vi "EITDATA_SubFunctions.vi"() -> ()   [LabVIEW 2020]
doc: "This example demonstrates how to acquire a single buffer of voltage measurements using a DAQmx device.\n\nFor instructions on how to connect your signals to the DAQ device, refer to your device documentation."
uses:
  <vilib>/Utility/error.llb/DialogType.ctl
  <vilib>/DAQmx/read.llb/DAQmx Read (Analog 1D Wfm NChan NSamp).vi
  <vilib>/DAQmx/create/channels.llb/DAQmx Create Channel (AI-Voltage-Basic).vi
  <vilib>/DAQmx/configure/timing.llb/DAQmx Timing (Sample Clock).vi
  <vilib>/DAQmx/configure/trigger.llb/DAQmx Start Trigger (Digital Edge).vi
  <vilib>/DAQmx/configure/trigger.llb/DAQmx Start Trigger (Time).vi
  <vilib>/DAQmx/configure/trigger.llb/DAQmx Start Trigger (Analog Edge).vi
  <vilib>/DAQmx/configure/trigger.llb/DAQmx Reference Trigger (Digital Edge).vi
  <vilib>/DAQmx/configure/trigger.llb/DAQmx Reference Trigger (Analog Edge).vi
  <vilib>/DAQmx/miscellaneous.llb/DAQmx Fill In Error Info.vi
  <vilib>/express/express analysis/Spectral/Block/exnSpectralBlock spectral measurements PSD poly.vi
  <vilib>/express/express analysis/Spectral/Block/exnSpectralBlock spectral measurements PSD array WFM.vi
  <vilib>/express/express analysis/Spectral/XNode/ExpressSpectralMeasurementsBlockNode.xnode
  <resource>/objmgr/daqmx.rc
panel:
  out "Waveform Chart 2":dbl[](graph)
  out "looptime":dbl
  out "Waveform Graph 3":dbl[][](graph)
  in  "header text must have # at startr":string="#header text header text texty text text"
  out "Waveform Chart":T1(graph)
  in  "name or relative path":string="test.txt"
  in  "stop":bool
  out "Waveform Graph 2":cluster{"f0":dbl, "df":dbl, "magnitude":dbl[]}[](graph)
  in  "Trigger Type":T2(tab)
  in  "Digital Start Trigger Edge":i32(ring)=10280 caption="Edge" items=["Rising"=10280, "Falling"=10171]
  in  "Digital Start Trigger Source":tag="/Dev3/PFI0" caption="Source"
  in  "Digital Pause Trigger Pause When":i32(ring)=10192 caption="Pause When" items=["High"=10192, "Low"=10214]
  in  "Digital Pause Trigger Source":tag="/Dev1/PFI0" caption="Source"
  in  "Digital Reference Trigger Source":tag="/Dev1/PFI0" caption="Source"
  in  "Digital Reference Trigger Edge":i32(ring)=10280 caption="Edge" items=["Rising"=10280, "Falling"=10171]
  in  "Digital Reference Pretrigger Samples":u32 caption="Pretrigger Samples"
  in  "Analog Start Trigger Level":dbl caption="Level" format="%0.2f"
  in  "Analog Start Trigger Hysteresis":dbl caption="Hysteresis" format="%.2f"
  in  "Analog Start Trigger Slope":i32(ring)=10280 caption="Slope" items=["Rising"=10280, "Falling"=10171]
  in  "Analog Start Trigger Source":string="APFI0" caption="Source"
  in  "Analog Pause Trigger Source":string="APFI0" caption="Source"
  in  "Analog Pause Trigger Pause When":i32(ring)=10093 caption="Pause When" items=["Above Level"=10093, "Below Level"=10107]
  in  "Analog Pause Trigger Level":dbl caption="Level" format="%.2f"
  in  "Analog Reference Trigger Source":string="APFI0" caption="Source"
  in  "Analog Reference Trigger Level":dbl caption="Level" format="%.2f"
  in  "Analog Reference Trigger Slope":i32(ring)=10280 caption="Slope" items=["Rising"=10280, "Falling"=10171]
  in  "Analog Reference Pretrigger Samples":u32 caption="Pretrigger Samples"
  in  "When":timestamp
  in  "Select Time\nManually":bool
  out "Waveform Graph":waveform(dbl)[](graph)
  in  "Number of Samples":i32=1000
  in  "Sample Rate":dbl=50000.0
  in  "Sample Clock Source":tag="OnboardClock"
  in  "Terminal Configuration":i32(ring)=10083 items=["default"=-1, "RSE"=10083, "NRSE"=10078, "Differential"=10106, "Pseudodifferential"=12529]
  in  "Max Voltage":dbl=1.0
  in  "Min Voltage":dbl=-1.0
  in  "Physical Channel":tag="Dev3/ai0:15"
  out "Actual Sample Rate":dbl=1000.0 format="%0.2f"
  # "TIMEOUT AFTERWARDS IS NORMAL!!!!"
  # "Channel Settings"
  # "Acquired Data"
  # "Timing Settings"
  # "Trigger Settings"
  # "To enable triggers, select a tab above, and configure the settings.\n\nNot all hardware supports all trigger types. Refer to your device documentation for more information."
  # "If time is not manually set, task will begin after 10 seconds"
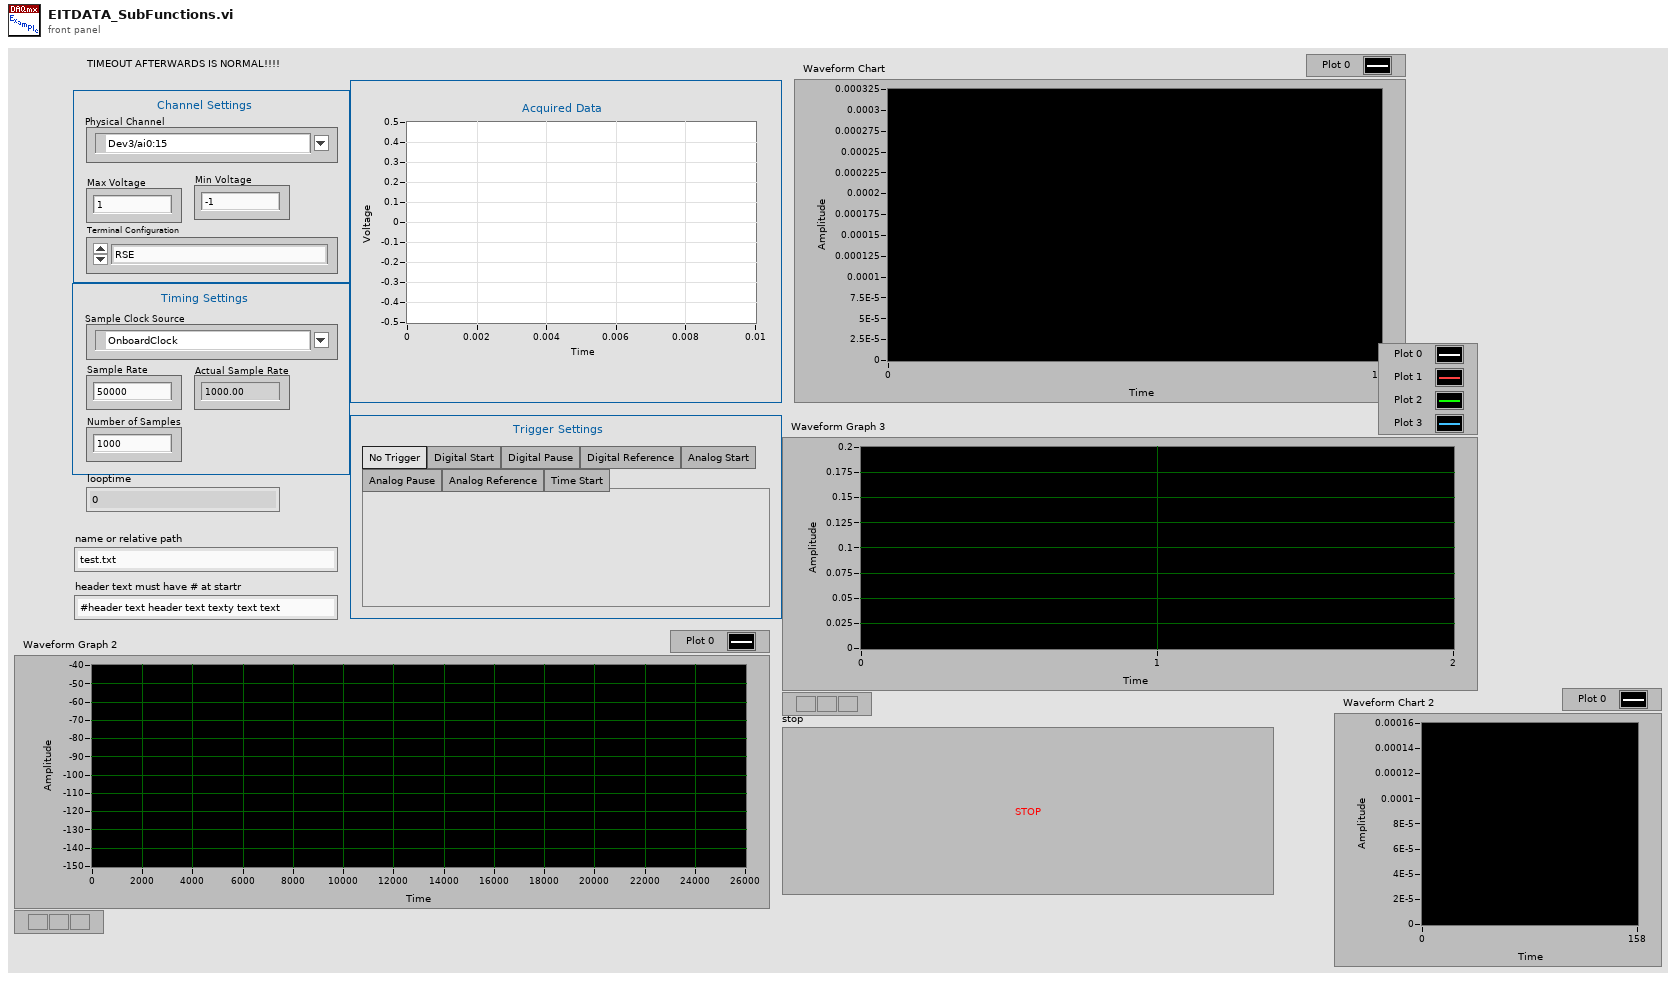
[diagram p1: front panel]
types:
  T1 = cluster{"detected amplitudes[0]":dbl, "detected amplitudes[1]":dbl, "detected amplitudes[2]":dbl, "detected amplitudes[3]":dbl, "detected amplitudes[4]":dbl, "detected amplitudes[5]":dbl, "detected amplitudes[6]":dbl, "detected amplitudes[7]":dbl, "detected amplitudes[8]":dbl}
  T2 = enum32{"No Trigger", "Digital Start", "Digital Pause", "Digital Reference", "Analog Start", "Analog Pause", "Analog Reference", "Time Start"}
  T3 = cluster{"detected amplitudes[0]":dbl, "detected amplitudes[1]":dbl, "detected amplitudes[2]":dbl, "detected amplitudes[3]":dbl, "detected amplitudes[4]":dbl, "detected amplitudes[5]":dbl, "detected amplitudes[6]":dbl, "detected amplitudes[7]":dbl, "detected amplitudes[8]":dbl}[]
  T4 = enum16{"open", "replace", "create", "open or create", "replace or create", "replace or create with confirmation"}
  T5 = typedef "DialogType.ctl" = u16
  T6 = cluster{"averaging mode":u16, "weighting mode":u16, "number of averages":u32}
  T7 = cluster{"dB On (F)":bool, "unwrap phase (F)":bool, "convert to degree (F)":bool}
  T8 = cluster{"Amp1D[0]":dbl, "Amp1D[1]":dbl, "Amp1D[2]":dbl, "Amp1D[3]":dbl, "Amp1D[4]":dbl, "Amp1D[5]":dbl, "Amp1D[6]":dbl, "Amp1D[7]":dbl, "Amp1D[8]":dbl}
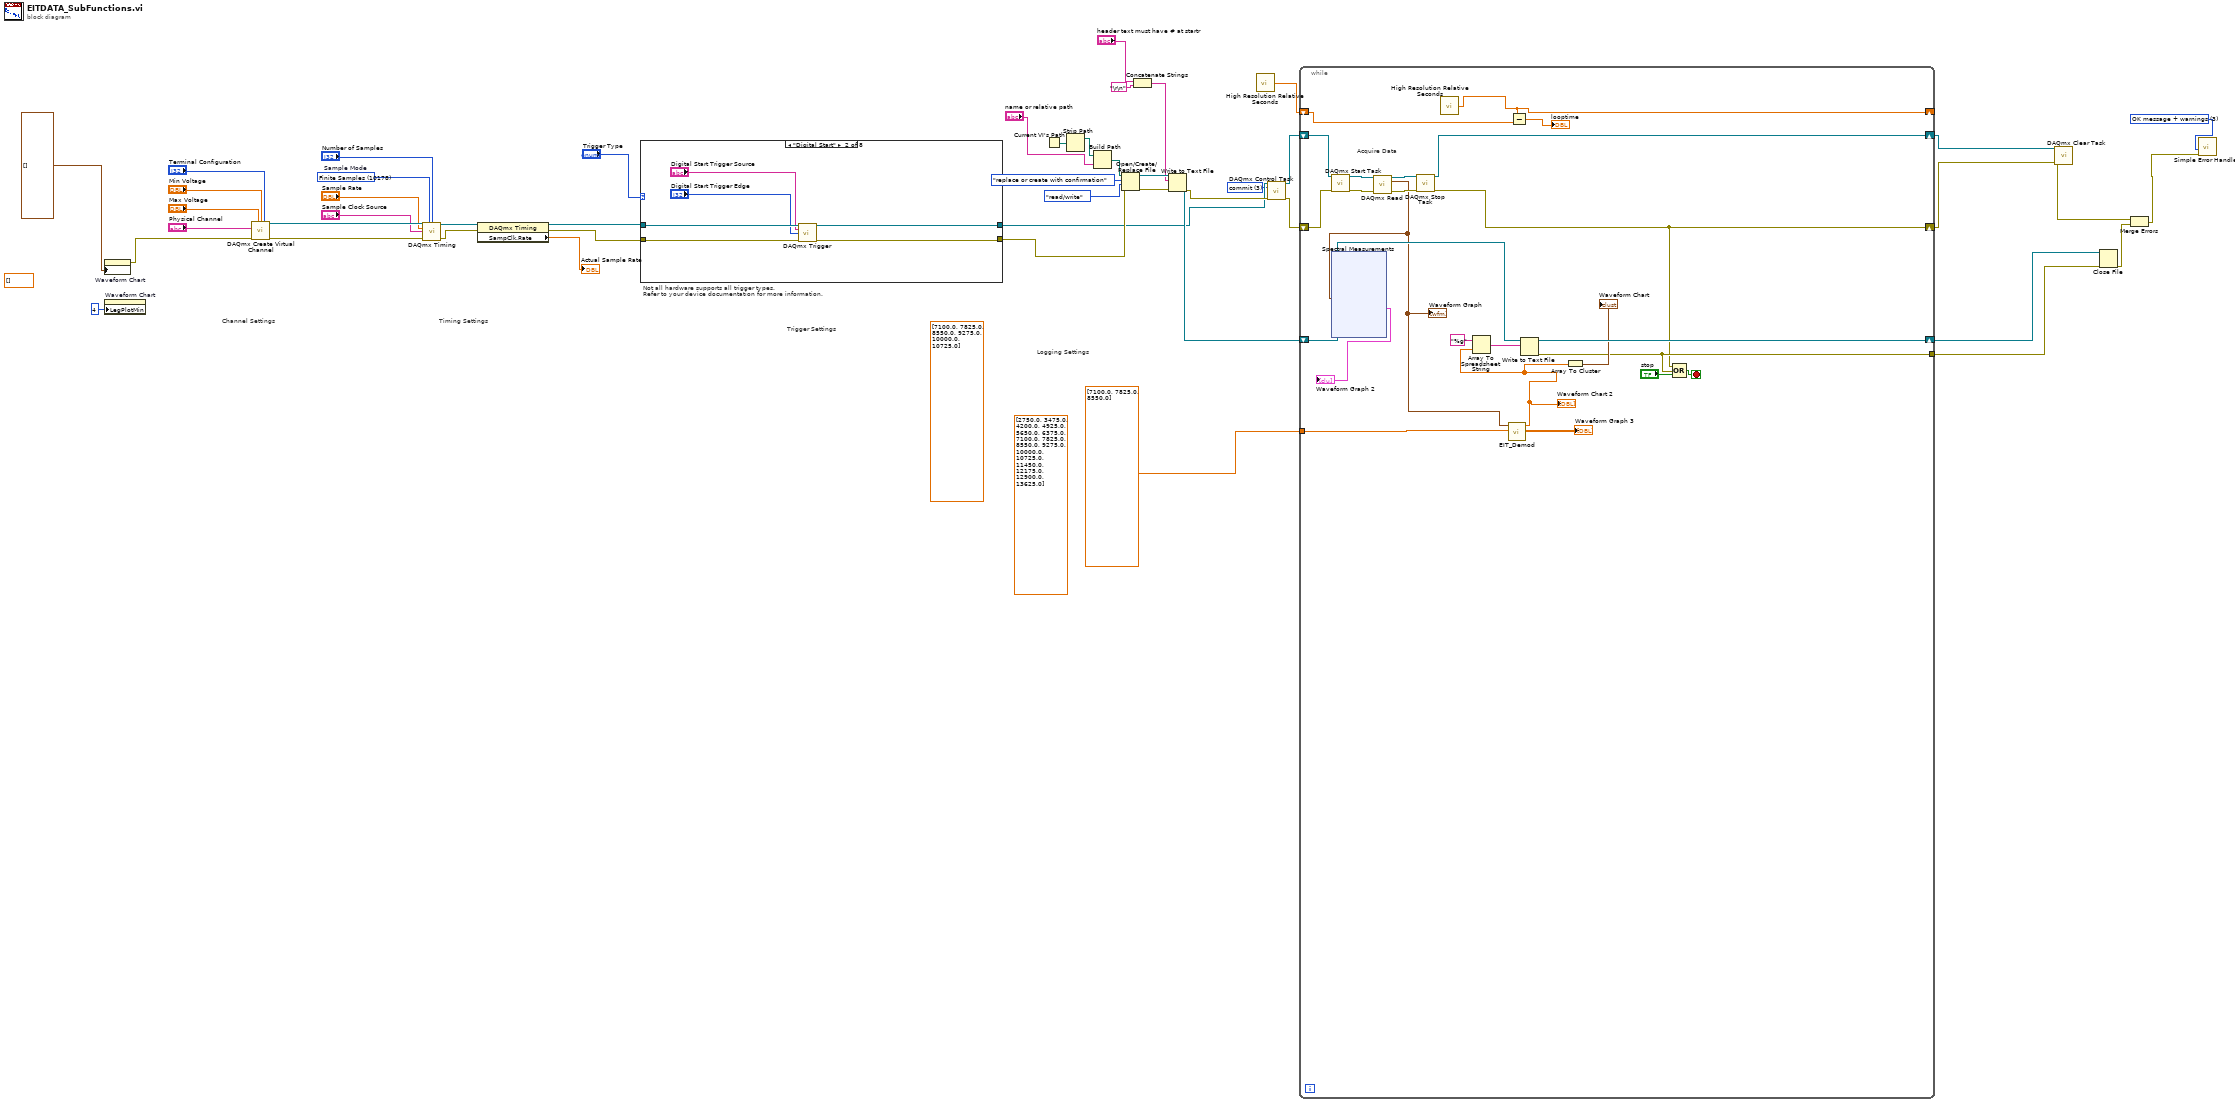
[diagram p0: block diagram]
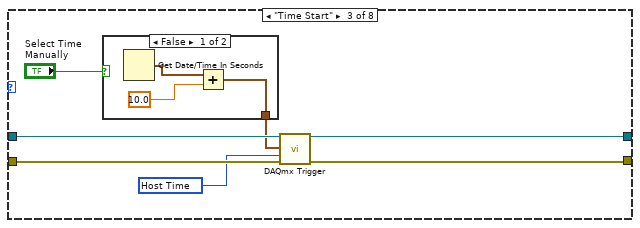
[diagram p3: hidden frame]
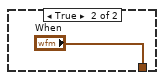
[diagram p4: hidden frame]
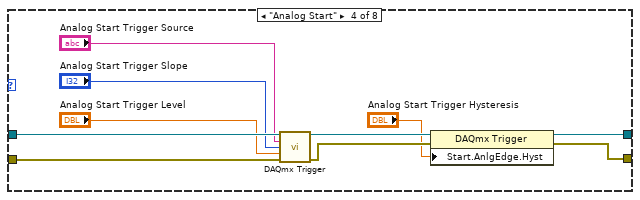
[diagram p5: hidden frame]
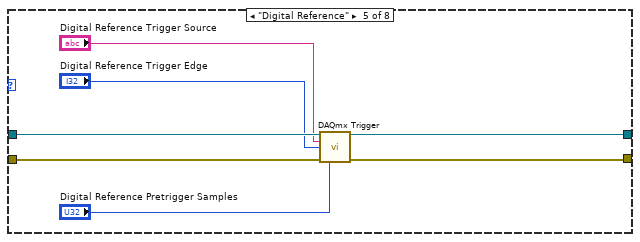
[diagram p6: hidden frame]
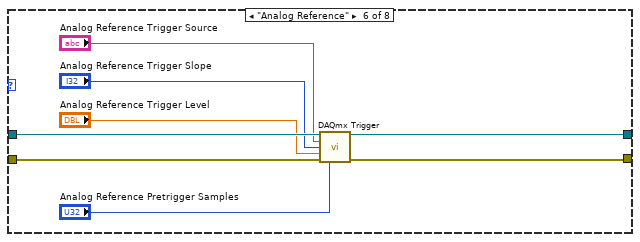
[diagram p7: hidden frame]
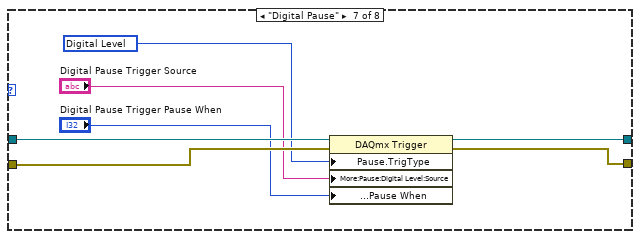
[diagram p8: hidden frame]
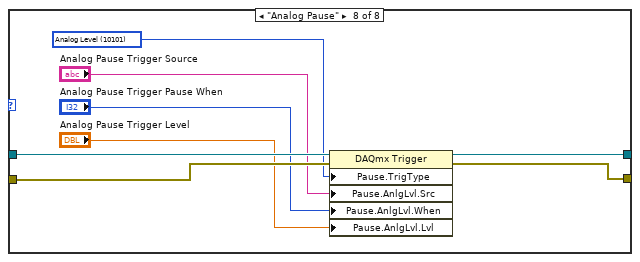
[diagram p9: hidden frame]
diagram:
  (unwired) dbl[] [7100.0, 7825.0, 8550.0, 9275.0, 10000.0, 10725.0]
  (unwired) dbl[] [2750.0, 3475.0, 4200.0, 4925.0, 5650.0, 6375.0, 7100.0, 7825.0, 8550.0, 9275.0, 10000.0, 10725.0, 11450.0, 12175.0, 12900.0, 13625.0]
  (unwired) dbl[] [] ("History Data")
  w12 = 3 items=["verify"=2, "reserve"=4, "commit"=3, "unreserve"=5, "abort"=6] ("action")
  w34 = T5 3 items=["no dialog", "OK message", "continue or stop message", "OK message + warnings", "continue/stop + warnings"] ("type of dialog (OK msg:1)")
  w45 = 10178 items=["Finite Samples"=10178, "Continuous Samples"=10123, "Hardware Timed Single Point"=12522]  # Sample Mode
  # "Not all hardware supports all trigger types.\nRefer to your device documentation for more information."
  # "Trigger Settings"
  # "Timing Settings"
  # "Channel Settings"
  # "Logging Settings"
  n1 = property on="Waveform Chart" class="WFChart (strict)"("History Data"=T3 []) -> (error out=w6:errorcluster)  [unwired: 2 in, 1 out]
  n2 = property on="Waveform Chart" class="WFChart (strict)"("LegPlotMin"=u32 4 ("Legend:Plot Minimum")) -> ()  [unwired: 2 in, 2 out]
  n3 = call-poly <vilib>:"DAQmx Create Virtual Channel.vi"("maximum value"="Max Voltage", "minimum value"="Min Voltage", "input terminal configuration"="Terminal Configuration", "physical channels"="Physical Channel", "error in"=w6) -> ("task out"=w43:refnum<k21>, "error out"=w44:errorcluster)  [unwired: 9 in]
  n4 = call-poly <vilib>:"DAQmx Timing.vi"("task/channels in"=w43, "sample mode"=w45, "samples per channel"="Number of Samples", "rate"="Sample Rate", "source"="Sample Clock Source", "error in"=w44) -> ("task out"=w47:refnum<k21>, "error out"=w46:errorcluster)  [unwired: 8 in]
  n5 = property class="DAQmx Timing"(reference=w47, error in=w46) -> (reference out=w31:refnum<k21>, error out=w32:errorcluster, "SampClk.Rate"=→"Actual Sample Rate":dbl)
  n6 = case shown="\"Digital Start\"" "Trigger Type" {
    tunnel: w31 -> [w49 w55 w62 w76 w83 w91 w98 w106]
    tunnel: w32 -> [w48 w54 w61 w75 w82 w90 w95 w103]
    tunnel: [w49 w53 w60 w73 w81 w89 w97 w105] -> w14
    tunnel: [w48 w52 w59 w72 w80 w88 w96 w104] -> w20
    frame "No Trigger", Default {
    }
    frame "Digital Start" {
      n7 = call-poly <vilib>:"DAQmx Trigger.vi"("task/channels in"=w55, "source"="Digital Start Trigger Source", "edge"="Digital Start Trigger Edge", "error in"=w54) -> ("task out"=w53:refnum<k21>, "error out"=w52:errorcluster)  [unwired: 10 in]
    }
    frame "Time Start" {
      w58 = 16126 items=["Host Time"=16126, "I/O Device Time"=16127] ("timescale")
      n8 = case shown="False" "Select Time\nManually" {
        tunnel: [w64 "When"] -> w56
        frame False {
          n9 = Get Date/Time In Seconds() -> (seconds since 1Jan1904=w65:timestamp)
          n10 = Add(x=w65, y=10.0) -> (x+y=w64:timestamp)
        }
        frame True {
        }
      }
      n11 = call-poly <vilib>:"DAQmx Trigger.vi"("task/channels in"=w62, "when"=w56, "timescale"=w58, "error in"=w61) -> ("task out"=w60:refnum<k21>, "error out"=w59:errorcluster)  [unwired: 10 in]
    }
    frame "Analog Start" {
      n12 = call-poly <vilib>:"DAQmx Trigger.vi"("task/channels in"=w76, "source"="Analog Start Trigger Source", "slope"="Analog Start Trigger Slope", "level"="Analog Start Trigger Level", "error in"=w75) -> ("task out"=w71:refnum<k21>, "error out"=w70:errorcluster)  [unwired: 9 in]
      n13 = property class="DAQmx Trigger"(reference=w71, error in=w70, "Start.AnlgEdge.Hyst"="Analog Start Trigger Hysteresis") -> (reference out=w73:refnum<k21>, error out=w72:errorcluster)
    }
    frame "Digital Reference" {
      n14 = call-poly <vilib>:"DAQmx Trigger.vi"("task/channels in"=w83, "source"="Digital Reference Trigger Source", "edge"="Digital Reference Trigger Edge", "error in"=w82, "pretrigger samples per channel"="Digital Reference Pretrigger Samples") -> ("task out"=w81:refnum<k21>, "error out"=w80:errorcluster)  [unwired: 9 in]
    }
    frame "Analog Reference" {
      n15 = call-poly <vilib>:"DAQmx Trigger.vi"("task/channels in"=w91, "source"="Analog Reference Trigger Source", "slope"="Analog Reference Trigger Slope", "level"="Analog Reference Trigger Level", "error in"=w90, "pretrigger samples per channel"="Analog Reference Pretrigger Samples") -> ("task out"=w89:refnum<k21>, "error out"=w88:errorcluster)  [unwired: 8 in]
    }
    frame "Digital Pause" {
      w94 = 10152 items=["Analog Level"=10101, "Analog Window"=10103, "Digital Level"=10152, "Digital Pattern"=10398, "None"=10230] ("Pause.TrigType")
      n16 = property class="DAQmx Trigger"(reference=w98, error in=w95, "Pause.TrigType"=w94, "More:Pause:Digital Level:Source"="Digital Pause Trigger Source", "More:Pause:Digital Level:Pause When"="Digital Pause Trigger Pause When") -> (reference out=w97:refnum<k21>, error out=w96:errorcluster)
    }
    frame "Analog Pause" {
      w102 = 10101 items=["Analog Level"=10101, "Analog Window"=10103, "Digital Level"=10152, "Digital Pattern"=10398, "None"=10230] ("Pause.TrigType")
      n17 = property class="DAQmx Trigger"(reference=w106, error in=w103, "Pause.TrigType"=w102, "Pause.AnlgLvl.Src"="Analog Pause Trigger Source", "Pause.AnlgLvl.When"="Analog Pause Trigger Pause When", "Pause.AnlgLvl.Lvl"="Analog Pause Trigger Level") -> (reference out=w105:refnum<k21>, error out=w104:errorcluster)
    }
  }
  n18 = Current VI's Path() -> (path=w25:path)
  n19 = Strip Path(path=w25) -> (stripped path=w19:path)  [unwired: 1 out]
  n20 = Build Path(base path=w19, name or relative path="name or relative path") -> (appended path=w28:path)
  n21 = Open/Create/Replace File(file path (use dialog)=w28, error in=w20, operation (0:open)=T4."replace or create with confirmation", access (0:read/write)=enum16{"read/write", "read-only", "write-only"}."read/write") -> (refnum out=w24:refnum<file>, error out=w23:errorcluster)  [unwired: 2 in, 1 out]
  n22 = Concatenate Strings("header text must have # at startr", "\r\n") -> (w22:string)
  n23 = Write to Text File(file (use dialog)=w24, text=w22, error in=w23) -> (refnum out=w17:refnum<file>, error out=w16:errorcluster)  [unwired: 1 in, 1 out]
  n24 = call <vilib>:"High Resolution Relative Seconds.vi"() -> ("relative seconds"=w2:dbl)
  n25 = call <vilib>:"DAQmx Control Task.vi"("task/channels in"=w14, "action"=w12, "error in"=w16) -> ("task out"=w13:refnum<k21>, "error out"=w15:errorcluster)  [unwired: 11 in]
  n26 = while {
    tunnel: [w115] -> w30
    shift-right: [w124] -> w29
    shift-left: w17 -> [w122]
    shift-right: [w114] -> w8
    shift-left: w15 -> [w121]
    shift-right: [w119] -> w11
    shift-left: w13 -> [w120]
    shift-right: [w112] -> _
    shift-left: w2 -> [w118]
    tunnel: dbl[] [7100.0, 7825.0, 8550.0] -> [w108]
    stop <- w113 stop-if-true
    # "Acquire Data"
    n27 = call <vilib>:"DAQmx Start Task.vi"("task/channels in"=w120, "error in"=w121) -> ("task out"=w130:refnum<k21>, "error out"=w129:errorcluster)  [unwired: 12 in]
    n28 = call-poly <vilib>:"DAQmx Read.vi"("task/channels in"=w130, "error in"=w129) -> ("task out"=w128:refnum<k21>, "data"=w110:waveform(dbl)[], "error out"=w127:errorcluster)  [unwired: 11 in]
    "Waveform Graph" <- w110
    n29 = xnode "Spectral Measurements"("Signals"=w110) -> ("PSD"=→"Waveform Graph 2":cluster{"f0":dbl, "df":dbl, "magnitude":dbl[]}[])  [unwired: 1 in, 1 out]
    n30 = call <vilib>:"DAQmx Stop Task.vi"("task/channels in"=w128, "error in"=w127) -> ("task out"=w119:refnum<k21>, "error out"=w114:errorcluster)  [unwired: 12 in]
    n31 = call <vilib>:"High Resolution Relative Seconds.vi"() -> ("relative seconds"=w112:dbl)
    n32 = call "EIT_Demod.vi"("Frequencies"=w108, "Waveforms"=w110) -> ("Amp2D"=→"Waveform Graph 3":dbl[][], "Amp1D"=w107:dbl[])  [unwired: 7 in, 1 out]
    "Waveform Chart 2" <- w107
    n33 = Array To Spreadsheet String(array=w107, 3:"%g" ("format string")) -> (spreadsheet string=w125:string)  [unwired: 1 in]
    n34 = Subtract(x=w112, y=w118) -> (x-y=→"looptime":dbl)
    n35 = Write to Text File(file (use dialog)=w122, text=w125) -> (refnum out=w124:refnum<file>, error out=w115:errorcluster)  [unwired: 2 in, 1 out]
    n36 = Array To Cluster(array=w107) -> (cluster=→"Waveform Chart":T8)
    n37 = Compound Arithmetic op=OR(w114, w115, "stop") -> (w113:bool)
  }
  n38 = call <vilib>:"DAQmx Clear Task.vi"("task in"=w11, "error in"=w8) -> ("error out"=w9:errorcluster)  [unwired: 13 in]
  n39 = Close File(refnum=w29, error in=w30) -> (error out=w10:errorcluster)  [unwired: 1 out]
  n40 = Merge Errors(w9, w10) -> (w18:errorcluster)
  n41 = call <vilib>:"Simple Error Handler.vi"("type of dialog (OK msg:1)"=w34, "error in (no error)"=w18) -> ()  [unwired: 3 in, 5 out]
